vi "Set_SN_Coords(openActiveX).vi"(8 "Coords EPOCH":dbl, 9 "input_DEC":dbl format="%<%H:%M:%S>t", 10 "input_RA":dbl format="%<%H:%M:%S%1u>t", 11 "ScopeSim._Telescope":refnum<k7>) -> (0 "precessed_DEC":dbl format="%<%H:%M:%S%1u>t", 3 "precessed_RA":dbl format="%<%H:%M:%S%2u>t")   [LabVIEW 2011]
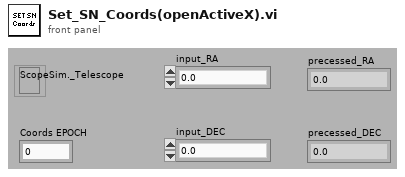
[diagram p1: front panel]
types:
  T1 = typedef "LVDateTimeRec.ctl" = cluster{"fractional second":dbl, "second":i32, "minute":i32, "hour":i32, "day of month":i32, "month":i32, "year":i32, "day of week":i32, "day of year":i32, "DST":i32}
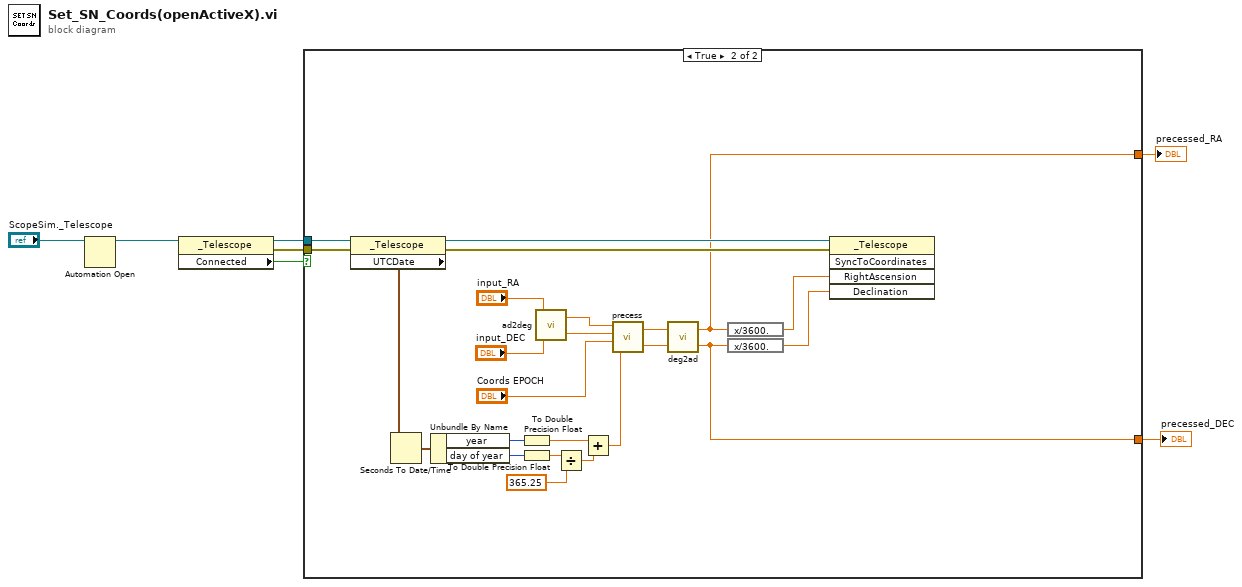
[diagram p0: block diagram]
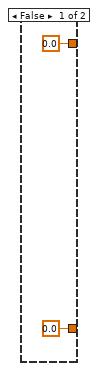
[diagram p2: hidden frame]
diagram:
  n1 = Automation Open(Automation Refnum="ScopeSim._Telescope") -> (Automation Refnum=w1:refnum<k7>)  [unwired: 3 in, 1 out]
  n2 = property class="_Telescope"(reference=w1) -> (reference out=w7:refnum<k7>, error out=w5:errorcluster, "Connected"=w6:bool)  [unwired: 1 in]
  n3 = case shown="True" w6 {
    tunnel: w7 -> [_ w33]
    tunnel: w5 -> [_ w23]
    tunnel: [0.0 ("RA (sec)") w10] -> w4
    tunnel: [0.0 ("DEC (sec)") w11] -> w3
    frame False {
    }
    frame True {
      n4 = property class="_Telescope"(reference=w33, error in=w23) -> (reference out=w25:refnum<k7>, error out=w22:errorcluster, "UTCDate"=w24:timestamp)
      n5 = Seconds To Date/Time(time stamp (now)=w24) -> (date time rec=w26:T1)  [unwired: 1 in]
      n6 = Unbundle By Name(w26) -> ("year"=w29:i32, "day of year"=w27:i32)
      n7 = To Double Precision Float(number=w29) -> (double precision float=w31:dbl)
      n8 = To Double Precision Float(number=w27) -> (double precision float=w28:dbl)
      n9 = call "ad2deg.vi"("DEC (sec)"="input_DEC", "RA (sec)"="input_RA") -> ("DEC (°)"=w18:dbl, "RA (°)"=w19:dbl)
      n10 = Divide(x=w28, y=365.25) -> (x/y=w32:dbl)
      n11 = Add(x=w31, y=w32) -> (x+y=w16:dbl)
      n12 = call "precess.vi"("Eq2"=w16, "Eq1"="Coords EPOCH", "DEC 1"=w18, "RA 1"=w19) -> ("DEC 2"=w15:dbl, "RA 2"=w14:dbl)
      n13 = call "deg2ad.vi"("DEC (°)"=w15, "RA (°)"=w14) -> ("DEC (°)"=w11:dbl, "RA (sec)"=w10:dbl)
      n14 = expression code="x/3600."(w10) -> (w12:dbl)
      n15 = expression code="x/3600."(w11) -> (w13:dbl)
      n16 = invoke class="_Telescope" method="SyncToCoordinates"(reference=w25, error in=w22, "RightAscension"=w12, "Declination"=w13) -> ()  [unwired: 1 in, 5 out]
    }
  }
  "precessed_RA" <- w4
  "precessed_DEC" <- w3
